vi "Update Script Body.vi"(8 "error in":errorcluster, 10 "Script UI Ctrl Ref":T2, 11 "Script Meas Config Ctrl Ref":T1) -> (0 "error out":errorcluster)   [LabVIEW 2025, in "Fgen Script Mode UI.lvlib"]
uses:
  Fgen Script Mode UI.lvlib
  Typedef/Script Meas Config Ctrl Ref.ctl
  Typedef/Script UI Ctrl Ref.ctl
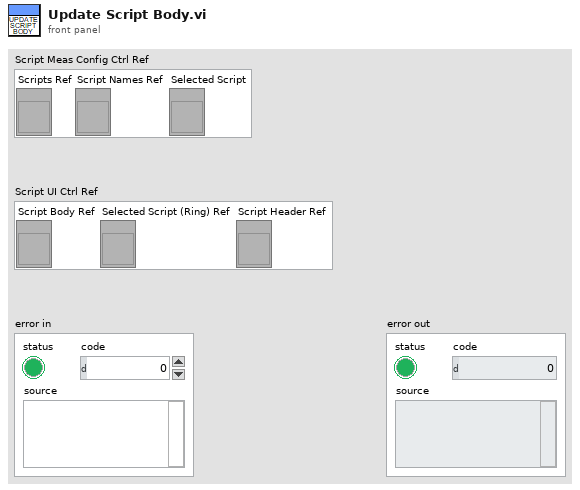
[diagram p1: front panel]
types:
  T1 = typedef "Fgen Script Mode UI.lvlib/Script Meas Config Ctrl Ref.ctl" = cluster{"Scripts Ref":refnum<vi>, "Script Names Ref":refnum<vi>, "Selected Script":refnum<vi>}
  T2 = typedef "Fgen Script Mode UI.lvlib/Script UI Ctrl Ref.ctl" = cluster{"Script Body Ref":refnum<vi>, "Selected Script (Ring) Ref":refnum<vi>, "Script Header Ref":refnum<vi>}
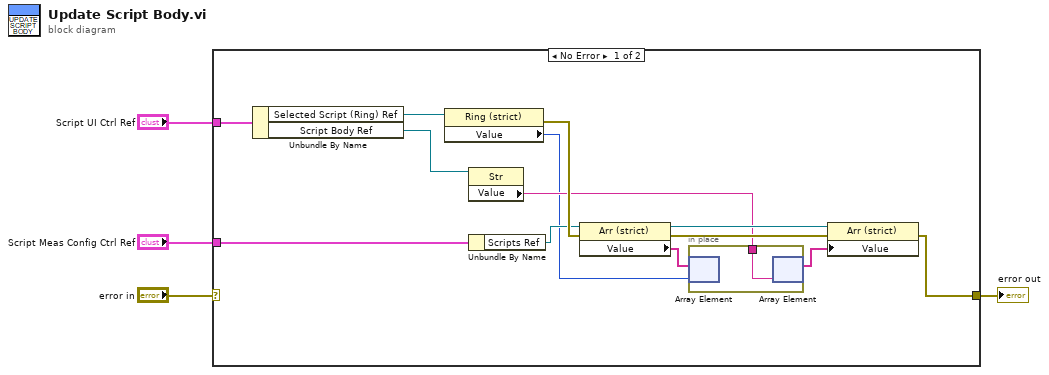
[diagram p0: block diagram]
diagram:
  n1 = case shown="No Error" "error in" {
    selector: "error in" -> [_ w19]
    tunnel: [w13 w19] -> w3
    tunnel: "Script Meas Config Ctrl Ref" -> [w11 _]
    tunnel: "Script UI Ctrl Ref" -> [w17 _]
    frame No Error {
      n2 = Unbundle By Name(w17) -> ("Selected Script (Ring) Ref"=w16:refnum<vi>, "Script Body Ref"=w9:refnum<vi>)
      n3 = property class="Ring (strict)"(reference=w16) -> (error out=w12:errorcluster, "Value"=w5:u16)  [unwired: 1 in, 1 out]
      n4 = property class="Str"(reference=w9) -> ("Value"=w7:string)  [unwired: 1 in, 2 out]
      n5 = Unbundle By Name(w11) -> ("Scripts Ref"=w10:refnum<vi>)
      n6 = property class="Arr (strict)"(reference=w10, error in=w12) -> (reference out=w15:refnum<vi>, error out=w14:errorcluster, "Value"=w8:string[])
      n7 = in-place {
        in-place-border: w7 -> [w18]
        n8 = in-place-array #1(w8, w5) -> ()  [unwired: 1 out]
        n9 = in-place-array #1(w18) -> (w6:string[])  [unwired: 1 out]
      }
      n10 = property class="Arr (strict)"(reference=w15, error in=w14, "Value"=w6) -> (error out=w13:errorcluster)  [unwired: 1 out]
    }
    frame Error {
    }
  }
  "error out" <- w3
